vi "set caption size.vi"(8 "error in (no error)":errorcluster, 9 "control visible":bool, 10 "Caption.Size":T1, 11 "Ctl Refnum in":refnum<vi>) -> (0 "error out":errorcluster, 3 "Ctl Refnum out":refnum<vi>)   [LabVIEW 2015, in "AguaClara Library.lvlib"]
uses:
  AguaClara Library.lvlib
  <vilib>/Utility/miscctls.llb/LVBoundsTypeDef.ctl
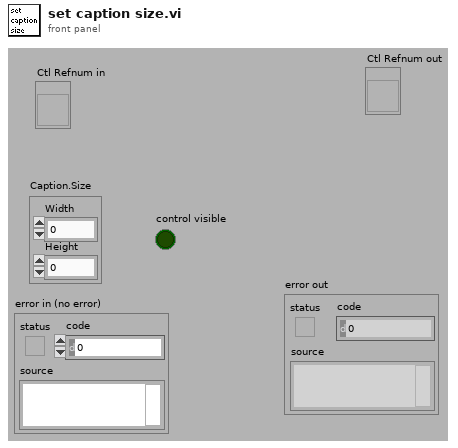
[diagram p1: front panel]
types:
  T1 = typedef "LVBoundsTypeDef.ctl" = cluster{"Width":u32, "Height":u32}
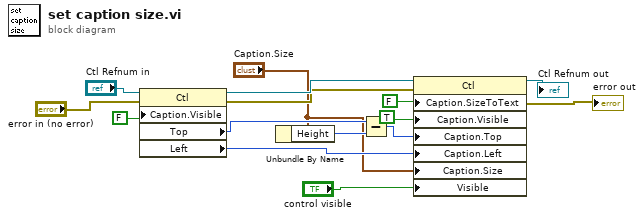
[diagram p0: block diagram]
diagram:
  n1 = property class="Ctl"(reference="Ctl Refnum in", error in="error in (no error)", "Caption.Visible"=FALSE) -> (reference out=w13:refnum<vi>, error out=w12:errorcluster, "Top"=w10:i32, "Left"=w8:i32)
  n2 = Unbundle By Name("Caption.Size") -> ("Height"=w15:u32)
  n3 = Subtract(x=w10, y=w15) -> (x-y=w9:u32)
  n4 = property class="Ctl"(reference=w13, error in=w12, "Caption.SizeToText"=FALSE ("Caption.Size to Text?"), "Caption.Visible"=TRUE, "Caption.Top"=w9, "Caption.Left"=w8, "Caption.Size"="Caption.Size", "Visible"="control visible") -> (reference out=→"Ctl Refnum out":refnum<vi>, error out=→"error out":errorcluster)
